vi "Window-8-bit Export-Output setup.vi"() -> (0 "error out (no error)":errorcluster)   [LabVIEW 2020]
uses:
  Global Variables/General Globals.vi
panel:
  in  "Frames Per Second":u32=30 min=1 max=1000 format="%.0f FPS"
  in  "Cancel":bool
  in  "OK":bool
  in  "Tab":enum32{"Setup", "Benchmarks A", "Benchmarks B"}(tab)
  in  "AVI mode":enum16{"AVI1", "AVI2"}(ring)=enum."AVI2"
  in  "Codec":u16(ring) items=["Intel IYUV codec", "Cinepak Codec by Radius", "Microsoft Video 1", "FF Video Codec 1 (FFV1) (NI Vision)", "Motion JPEG (NI Vision)", "Y800 Uncompressed Grey Scale (NI Vision)", "YUV 4:2:0 Planar (NI Vision)"]
  # "Set the desired frame-rate for the output video."
  # "AVI1: Lesser quality, slower, unlimited file size, opens in whiskers tracker.\nAVI2: Best quality, fast, generates 2GB split files."
  # "Choose a compression codec. Codecs are compression decoders each offering different image quality and file compression characteristics."
  # "3 seconds of 512x512 timelapse + 1 bodycam image"
  # "3 seconds of 512x512 timelapse + 3 bodycam images"
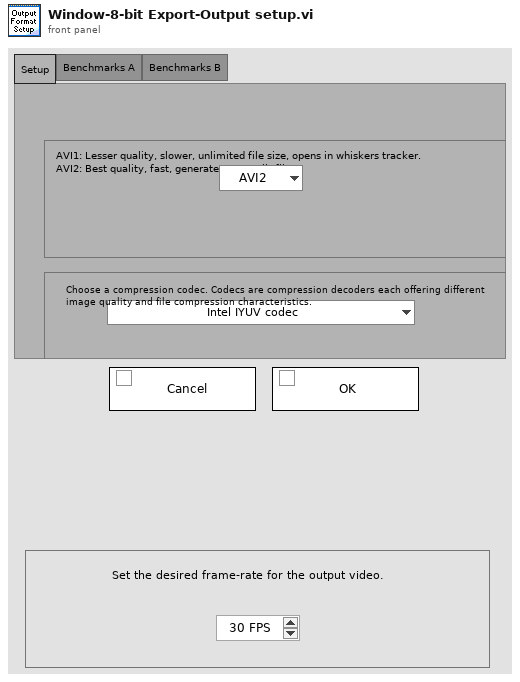
[diagram p1: front panel]
types:
  T1 = typedef "AVI implementation enum.ctl" = enum16{"AVI1", "AVI2"}
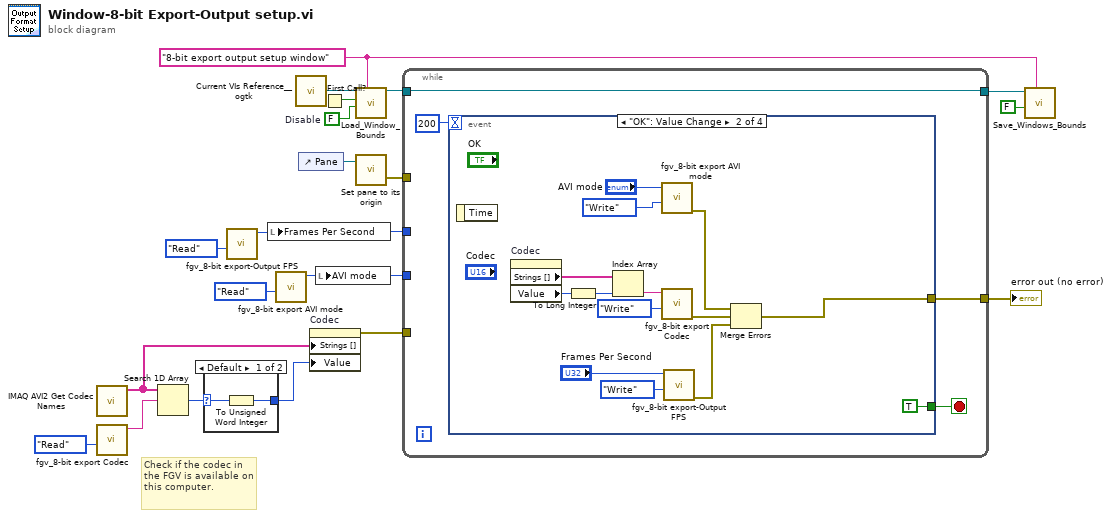
[diagram p0: block diagram]
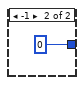
[diagram p2: hidden frame]
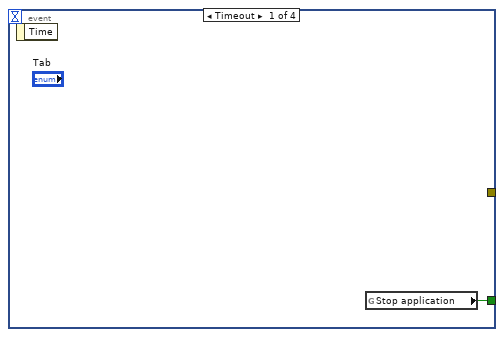
[diagram p3: hidden frame]
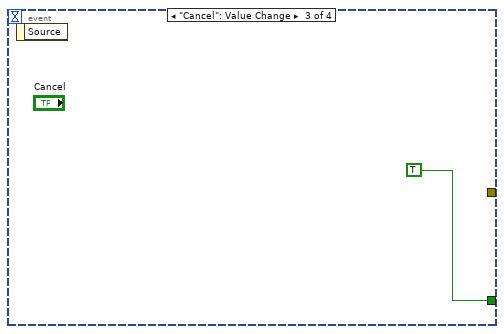
[diagram p4: hidden frame]
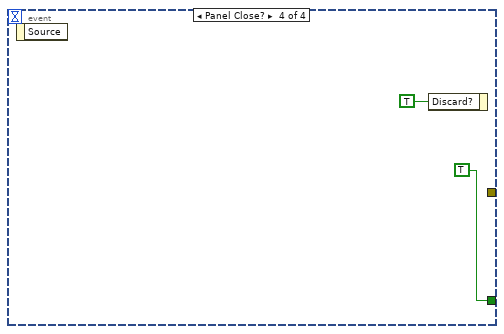
[diagram p5: hidden frame]
diagram:
  w16 = FALSE  # Disable
  w15 = "8-bit export output setup window" ("Window Name (i.e. Key)")
  # "Check if the codec in the FGV is available on this computer."
  n1 = call "IMAQ AVI2 Get Codec Names"() -> ("Codec Names"=w6:string[])  [unwired: 10 in, 1 out]
  n2 = call "fgv_8-bit export Codec.vi"("Function"=enum16{"Intialize", "Write", "Read", "Clear"}."Read") -> ("AVI mode"=w8:string)  [unwired: 9 in, 1 out]
  n3 = Search 1D Array(1D array=w6, element=w8) -> (index of element=w7:i32)  [unwired: 1 in]
  n4 = case shown="Default" w7 {
    selector: w7 -> [w22 _]
    tunnel: [w21 u16 0 ("index of element")] -> w5
    frame Default {
      n5 = To Unsigned Word Integer(number=w22) -> (unsigned 16bit integer=w21:u16)
    }
    frame -1 {
    }
  }
  n6 = call "fgv_8-bit export-Output FPS.vi"("Function"=enum16{"Intialize", "Write", "Read", "Clear"}."Read") -> ("Frames Per Second"=w2:u32)  [unwired: 9 in, 1 out]
  n7 = local write "Frames Per Second"(w2) -> ()
  n8 = call "fgv_8-bit export AVI mode.vi"("Function"=enum16{"Intialize", "Write", "Read", "Clear"}."Read") -> ("AVI mode"=w10:T1)  [unwired: 9 in, 1 out]
  n9 = call <userlib>:"Current VIs Reference__ogtk.vi"() -> ("Current VI's reference"=w18:refnum<vi>)  [unwired: 5 in]
  n10 = control-ref of="Pane"() -> (w20:refnum<vi>)
  n11 = property on="Codec" class="Ring (strict)"("Strings []"=w6, "Value"=w5) -> (error out=w4:errorcluster)  [unwired: 2 in, 1 out]
  n12 = local write "AVI mode"(w10) -> ()
  n13 = First Call?() -> (First Call?: T/F=w17:bool)
  n14 = call "Load_Window_Bounds.vi"("Window Name (i.e. Key)"=w15, "Disable"=w16, "First Call"=w17, "Window VI's Ref"=w18) -> ("reference out"=w12:refnum<vi>)  [unwired: 4 in, 3 out]
  n15 = call <userlib>:"Set pane to its origin.vi"("Pane Reference"=w20) -> ("error out (no error)"=w19:errorcluster)  [unwired: 9 in, 1 out]
  n16 = while {
    tunnel: w19 -> [_]
    tunnel: w12 -> [w26]
    tunnel: [w26] -> w13
    tunnel: w10 -> [_]
    tunnel: w4 -> [_]
    tunnel: w2 -> [_]
    tunnel: [w24] -> w1
    stop <- w27 stop-if-true
    n17 = event shown="[1] \"OK\": Value Change" {
      selector: _ -> [_ _ _ _]
      dyn-events: _ -> [_ _ _ _]
      timeout: 200 -> [_ _ _ _]
      tunnel: [w28 TRUE TRUE TRUE] -> w27
      tunnel: [_ w29 _ _] -> w24
      event Timeout {
        n18 = event-data() -> ()  [unwired: 1 in, 1 out]
        n19 = global read "General Globals.vi" "Stop application"() -> (w28:bool)
      }
      event "OK": Value Change {
        n20 = event-data() -> ()  [unwired: 1 in, 1 out]
        n21 = property on="Codec" class="Ring (strict)"() -> ("Strings []"=w37:string[], "Value"=w36:u16)  [unwired: 2 in, 2 out]
        n22 = To Long Integer(number=w36) -> (32bit integer=w35:i32)
        n23 = Index Array(array=w37, index=w35) -> (element=w39:string)
        n24 = call "fgv_8-bit export AVI mode.vi"("Function"=enum16{"Intialize", "Write", "Read", "Clear"}."Write", "AVI mode"="AVI mode") -> ("error out"=w32:errorcluster)  [unwired: 8 in, 1 out]
        n25 = call "fgv_8-bit export Codec.vi"("Function"=enum16{"Intialize", "Write", "Read", "Clear"}."Write", "Codec"=w39) -> ("error out"=w31:errorcluster)  [unwired: 8 in, 1 out]
        n26 = call "fgv_8-bit export-Output FPS.vi"("Function"=enum16{"Intialize", "Write", "Read", "Clear"}."Write", "Frames Per Second"="Frames Per Second") -> ("error out"=w30:errorcluster)  [unwired: 8 in, 1 out]
        n27 = Merge Errors(w32, w31, w30) -> (w29:errorcluster)
      }
      event "Cancel": Value Change {
        n28 = event-data() -> ()  [unwired: 1 in, 1 out]
      }
      event Panel Close? {
        n29 = event-data() -> ()  [unwired: 1 in, 1 out]
        n30 = event-data("Discard?"=TRUE) -> ()  [unwired: 1 in, 1 out]
      }
    }
  }
  "error out (no error)" <- w1
  n31 = call "Save_Windows_Bounds.vi"("Window Name (i.e. Key)"=w15, "Front Panel Window:Open"=FALSE, "Window VI's Ref"=w13) -> ()  [unwired: 8 in, 1 out]
